vi "Write AG.lvclass.vi"(8 "error in (no error)":errorcluster, 10 "AG.lvclass":refnum<class "AG.lvclass">, 11 "GuiderSetup in":refnum<class "GuiderSetup.lvclass">) -> (0 "error out":errorcluster, 3 "GuiderSetup out":refnum<class "GuiderSetup.lvclass">)   [LabVIEW 2018, in "GuiderSetup.lvclass"]
uses:
  GuiderSetup.lvclass
  AG/AG.lvclass
  GuiderSetup.lvclass/GuiderSetup.ctl
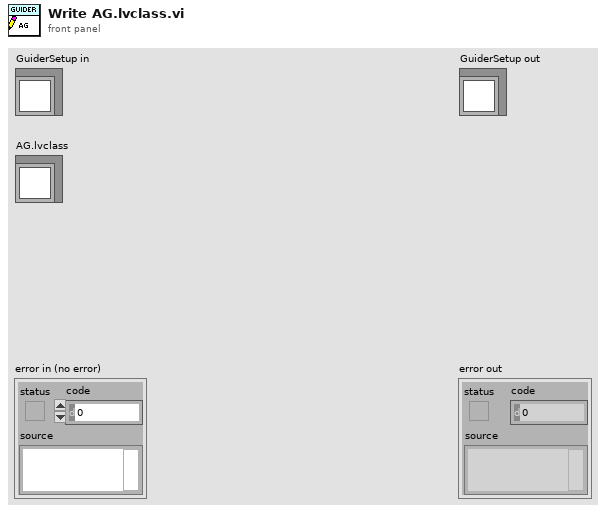
[diagram p1: front panel]
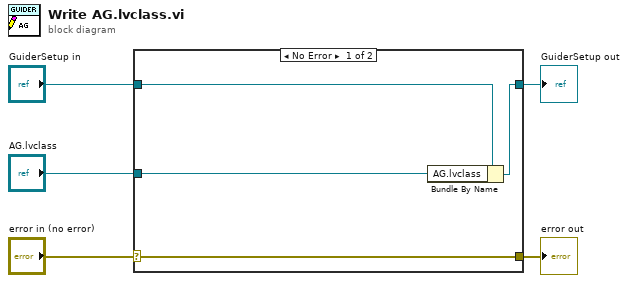
[diagram p0: block diagram]
diagram:
  n1 = case shown="No Error" "error in (no error)" {
    selector: "error in (no error)" -> [w9 w10]
    tunnel: [w9 w10] -> w4
    tunnel: [w7 w11] -> w2
    tunnel: "GuiderSetup in" -> [w8 w11]
    tunnel: "AG.lvclass" -> [w6 _]
    frame No Error {
      n2 = Bundle By Name(cluster=w8, "AG.lvclass"=w6) -> (w7:refnum<class "GuiderSetup.lvclass">)
    }
    frame Error {
    }
  }
  "error out" <- w4
  "GuiderSetup out" <- w2
